vi "save.vi"(8 "error in (no error)":errorcluster, 9 "base name":string, 10 "folder path":path, 11 "DL090215DataCollection in":refnum<class "DataCollectionMG091001IntrinsicImaging.lvclass">) -> (0 "error out":errorcluster, 3 "DL090215DataCollection out":refnum<class "DataCollectionMG091001IntrinsicImaging.lvclass">)   [LabVIEW 2010, in "DataCollectionMG091001IntrinsicImaging.lvclass"]
uses:
  DataCollectionMG091001IntrinsicImaging.lvclass
  sweep_part_enum.ctl
  DataCollectionDL091104Scaffold/DataCollectionDL091104Scaffold/DataCollectionDL091104Scaffold.lvclass
  common/classes/ErrorController/ErrorController/ErrorController.lvclass
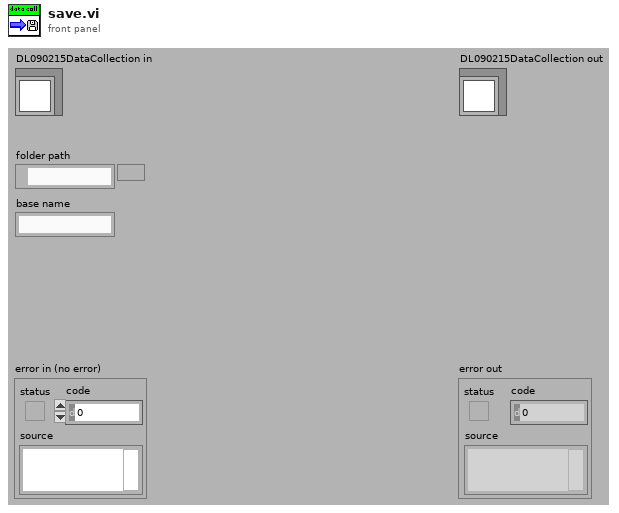
[diagram p1: front panel]
types:
  T1 = typedef "DataCollectionMG091001IntrinsicImaging.lvclass/average_save_type_enum.ctl" = enum16{"time course", "time average", "time course and average"}
  T2 = enum16{"time course", "time average", "time course and average"}[]
  T3 = typedef "DataCollectionMG091001IntrinsicImaging.lvclass/sweep_part_enum.ctl" = enum16{"actual measurement", "control"}
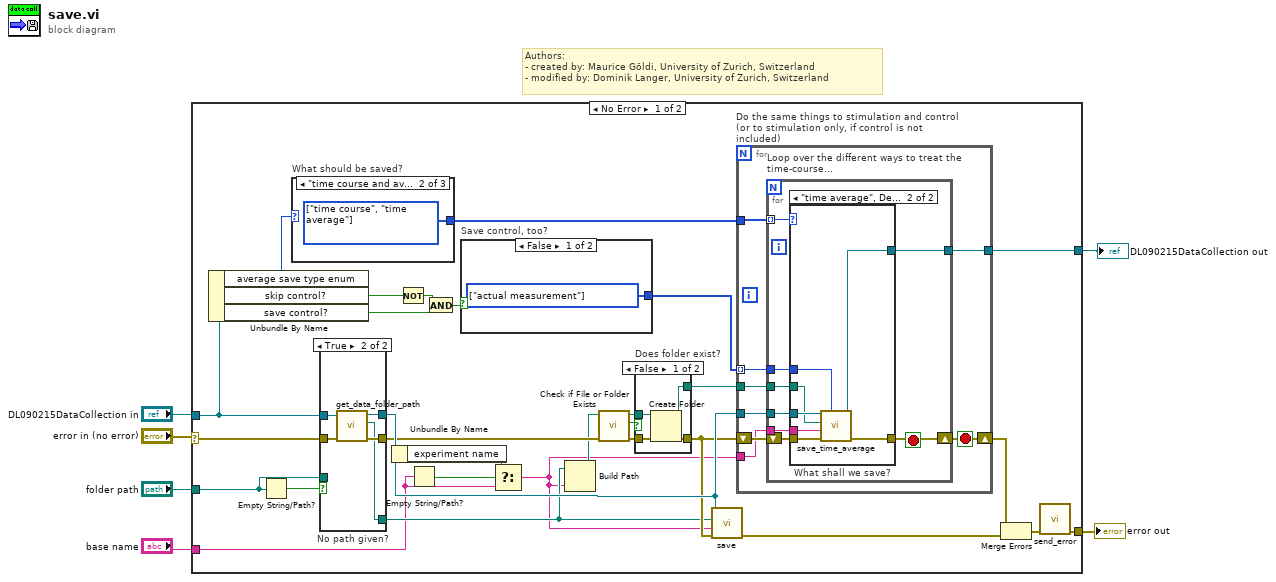
[diagram p0: block diagram]
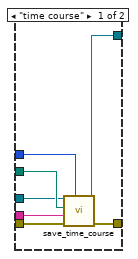
[diagram p4: hidden frame]
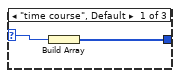
[diagram p5: hidden frame]
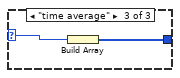
[diagram p6: hidden frame]
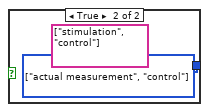
[diagram p7: hidden frame]
diagram:
  # "Authors: \n- created by: Maurice Göldi, University of Zurich, Switzerland\n- modified by: Dominik Langer, University of Zurich, Switzerland"
  n1 = case shown="No Error" "error in (no error)" {
    selector: "error in (no error)" -> [w8 w88]
    tunnel: [w23 w88] -> w5
    tunnel: "DL090215DataCollection in" -> [w19 w87]
    tunnel: [w20 w87] -> w4
    tunnel: "folder path" -> [w26 _]
    tunnel: "base name" -> [w12 _]
    frame No Error {
      n2 = Unbundle By Name(w19) -> ("average save type enum"=w35:T1, "skip control?"=w33:bool, "save control?"=w31:bool)
      n3 = Empty String/Path?(string/path=w26) -> (empty?=w27:bool)
      n4 = case "What should be saved?" shown="\"time course and average\"" w35 {
        selector: w35 -> [w81 _ w83]
        tunnel: [w80 w82 w84] -> w34
        frame "time course", Default {
          n5 = Build Array(w81) -> (w80:T1[])
        }
        frame "time course and average" {
          w82 = T2 [enum."time course", enum."time average"] items=["time course", "time average", "time course and average"]
        }
        frame "time average" {
          n6 = Build Array(w83) -> (w84:T1[])
        }
      }
      n7 = case "No path given?" shown="True" w27 {
        tunnel: [w42 w49] -> w18
        tunnel: [w44 w48] -> w29
        tunnel: w8 -> [w42 w47]
        tunnel: w19 -> [w44 w46]
        tunnel: [w43 w45] -> w21
        tunnel: w26 -> [w43 _]
        frame False {
        }
        frame True {
          n8 = call-dynamic "get_data_folder_path.vi"("error in (no error)"=w47, "GenericComponent in"=w46) -> ("error out"=w49:errorcluster, "data folder path"=w45:path, "GenericComponent out"=w48:refnum<class "DataCollectionMG091001IntrinsicImaging.lvclass">)  [unwired: 7 in]
        }
      }
      n9 = Unbundle By Name(w29) -> ("experiment name"=w10:string)
      n10 = Not(x=w33) -> (.not. x?=w32:bool)
      n11 = Empty String/Path?(string/path=w12) -> (empty?=w11:bool)
      n12 = And(x=w32, y=w31) -> (x .and. y?=w30:bool)
      n13 = case "Save control, too?" shown="False" w30 {
        tunnel: [w85 w86] -> w25
        frame False {
          w85 = T3[] [enum."actual measurement"] items=["actual measurement", "control"]
        }
        frame True {
          w86 = T3[] [enum."actual measurement", enum."control"] items=["actual measurement", "control"]
          (unwired) string[] ["stimulation", "control"]
        }
      }
      n14 = Select(t=w10, s=w11, f=w12) -> (s? t:f=w9:string)
      n15 = Build Path(base path=w21, name or relative path=w9) -> (appended path=w16:path)
      n16 = call <vilib>:"Check if File or Folder Exists.vi"("error in (no error)"=w18, "path"=w16) -> ("error out"=w17:errorcluster, "file or folder exists?"=w13:bool, "dup path"=w15:path)  [unwired: 7 in]
      n17 = case "Does folder exist?" shown="False" w13 {
        tunnel: [w39 w40] -> w22
        tunnel: w17 -> [w38 w40]
        tunnel: w15 -> [w37 w41]
        tunnel: [w36 w41] -> w14
        frame False {
          n18 = Create Folder(path (use dialog)=w37, error in=w38) -> (created path=w36:path, error out=w39:errorcluster)  [unwired: 1 in, 1 out]
        }
        frame True {
        }
      }
      n19 = call-parent "save.vi"("error in (no error)"=w22, "base name"=w9, "folder path"=w21, "DL090215DataCollection in"=w29) -> ("error out"=w28:errorcluster)  [unwired: 6 in, 1 out]
      n20 = for "Do the same things to stimulation and control (or to stimulation only, if control is not included)" {
        tunnel: [w52] -> w20
        tunnel: w29 -> [w55]
        tunnel: w9 -> [w53]
        tunnel: w14 -> [w54]
        tunnel: w34 -> [w57]
        tunnel: w25 -> [w51] mode=indexing
        shift-right: [w50] -> w7
        shift-left: w22 -> [w56]
        stop <- w50 stop-if-true
        n21 = for "Loop over the different ways to treat the time-course..." {
          tunnel: [w64] -> w52
          tunnel: w55 -> [w63]
          tunnel: w57 -> [w62] mode=indexing
          tunnel: w53 -> [w61]
          tunnel: w54 -> [w60]
          tunnel: w51 -> [w59]
          shift-right: [w58] -> w50
          shift-left: w56 -> [w65]
          stop <- w58 stop-if-true
          n22 = case "What shall we save?" shown="\"time average\", Default" w62 {
            tunnel: [w67 w74] -> w58
            tunnel: w65 -> [w72 w79]
            tunnel: [w68 w73] -> w64
            tunnel: w63 -> [w70 w77]
            tunnel: w61 -> [w69 w78]
            tunnel: w60 -> [w71 w75]
            tunnel: w59 -> [w66 w76]
            frame "time course" {
              n23 = call-dynamic "save_time_course.vi"("stimulation type enum"=w66, "error in (no error)"=w72, "base name"=w69, "folder path"=w71, "DataCollectionMG091001IntrinsicImaging in"=w70) -> ("error out"=w67:errorcluster, "DataCollectionMG091001IntrinsicImaging out"=w68:refnum<class "DataCollectionMG091001IntrinsicImaging.lvclass">)  [unwired: 5 in]
            }
            frame "time average", Default {
              n24 = call-dynamic "save_time_average.vi"("stimulation type enum"=w76, "error in (no error)"=w79, "base name"=w78, "folder path"=w75, "DataCollectionMG091001IntrinsicImaging in"=w77) -> ("error out"=w74:errorcluster, "DataCollectionMG091001IntrinsicImaging out"=w73:refnum<class "DataCollectionMG091001IntrinsicImaging.lvclass">)  [unwired: 5 in]
            }
          }
        }
      }
      n25 = Merge Errors(w7, w28) -> (w24:errorcluster)
      n26 = call "send_error.vi"("error in (no error)"=w24) -> ("error out"=w23:errorcluster)  [unwired: 10 in]
    }
    frame Error {
    }
  }
  "error out" <- w5
  "DL090215DataCollection out" <- w4
